vi "ui_read_stream_from_rt.vi"(11 "Message Queue":refnum<queue> caption="消息队列") -> (0 "error out":errorcluster caption="错误输出", 2 "Message Received?":bool caption="收到消息？", 3 "dup Message Queue":refnum<queue> caption="消息队列副本")   [LabVIEW 2015]
uses:
  message_queue/message_cluster.ctl
  globals/global_ui_stream_and_variable_connections.vi
  message_queue/message_queue.lvlib
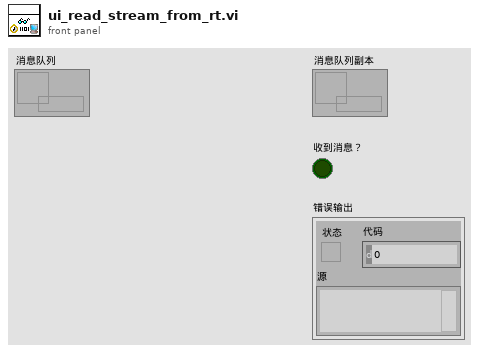
[diagram p1: front panel]
types:
  T1 = typedef "Message Queue.lvlib/Message Cluster.ctl" = cluster{"Message":string, "Message Data":variant}
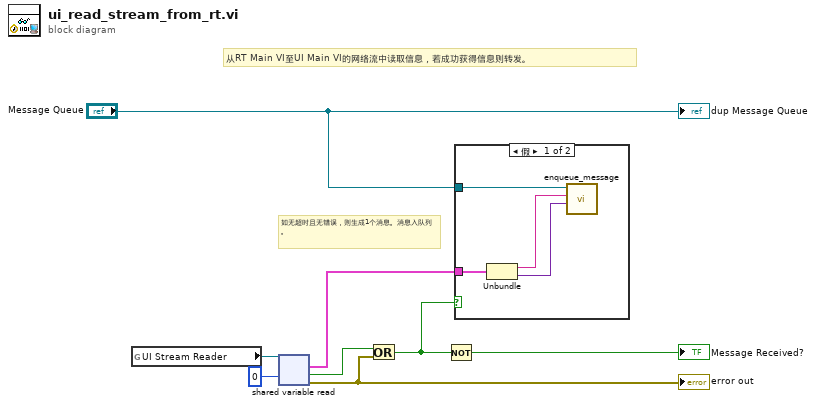
[diagram p0: block diagram]
diagram:
  # "如无超时且无错误，则生成1个消息。消息入队列。"
  # "从RT Main VI至UI Main VI的网络流中读取信息，若成功获得信息则转发。"
  n1 = global read "global_ui_stream_and_variable_connections.vi" "UI Stream Reader"() -> (w4:refnum<k21>)
  n2 = shared-variable-read(w4, 0 ("timeout ms (-1)")) -> (w6:errorcluster, w8:bool, w7:T1)  [unwired: 1 in, 1 out]
  "error out" <- w6
  n3 = Or(x=w8, y=w6) -> (x .or. y?=w3:bool)
  n4 = Not(x=w3) -> (.not. x?=→"Message Received?":bool)
  n5 = case shown="假" w3 {
    tunnel: w7 -> [w11 _]
    tunnel: "Message Queue" -> [w12 _]
    frame False {
      n6 = Unbundle(w11) -> ("Message"=w10:string, "Message Data"=w9:variant)
      n7 = call "enqueue_message.vi"("Message Data"=w9, "Message"=w10, "Message Queue"=w12) -> ()  [unwired: 7 in, 2 out]
    }
    frame True {
    }
  }
  "dup Message Queue" <- "Message Queue"
